vi "Linda_CORE_svi_FGV.vi"(1 "OP":T1, 5 "IN VARIANT":variant, 9 "Name in":string, 11 "error in (no error)":errorcluster, 12 "Space size":i32=1000000) -> (4 "Number of  Tuples":i32, 6 "OUT VARIANT":variant, 8 "Rd_all Array":variant[](array[variant]), 10 "Valid Op":bool, 15 "error out":errorcluster)   [LabVIEW 2015]
uses:
  LI_states.ctl
  C:/Users/Giuseppe/Downloads/LabLinda_ pakage/index_datatype.ctl
  C:/Users/Giuseppe/Downloads/LabLinda_ pakage/index_cluster.ctl
  index_datatype.ctl
  index_cluster.ctl
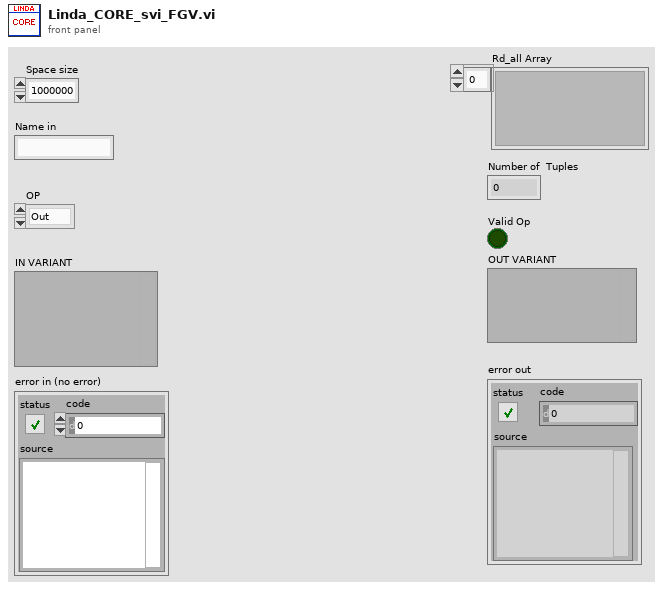
[diagram p1: front panel]
types:
  T1 = typedef "LI_states.ctl" = enum16{"Out", "In", "Rd", "Inp", "Rdp", "Init", "Cleanup", "RdAll"}
  T2 = enum16{"Init", "Read addr", "Write item", "Cleanup", "Add free", "Query Free"}
  T3 = enum32{"Invalid", "Standard", "Closed", "Hidden", "Minimized", "Maximized"}
  T4 = typedef "index_datatype.ctl" = T5[]
  T5 = typedef "index_cluster.ctl" = cluster{"Addr":i32[], "out react vi reference":refnum<vi>, "in react vi reference":refnum<vi>, "rd react vi reference":refnum<vi>, "Read_write_var":refnum<vi>}
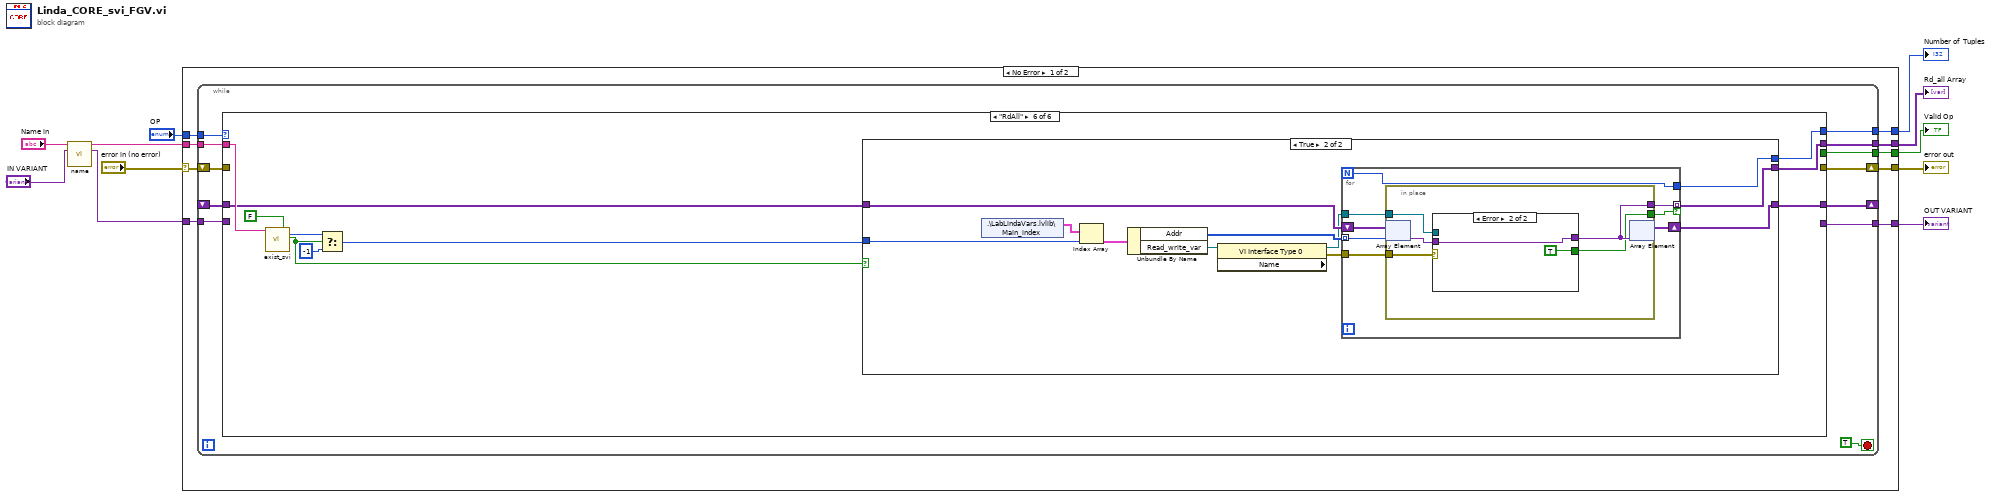
[diagram p0: block diagram]
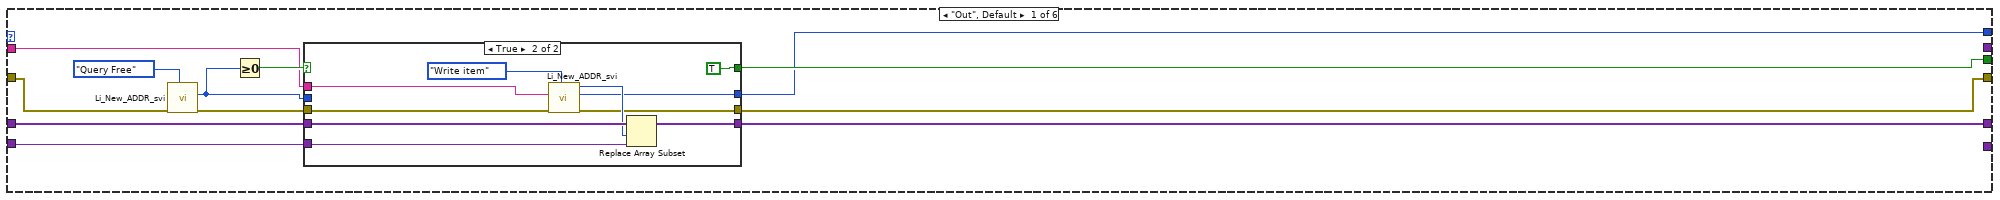
[diagram p2: hidden frame]
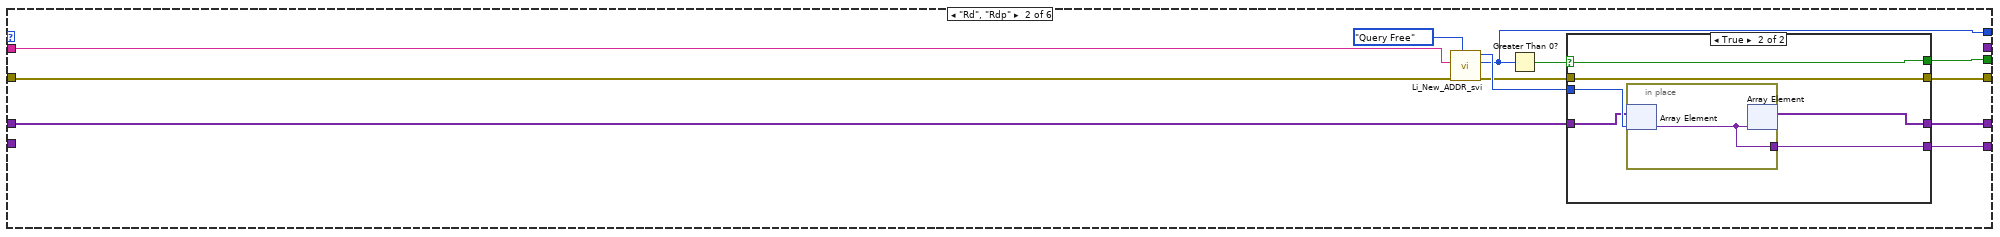
[diagram p4: hidden frame]
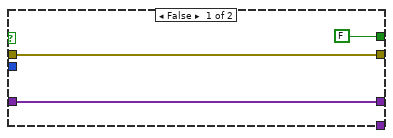
[diagram p5: hidden frame]
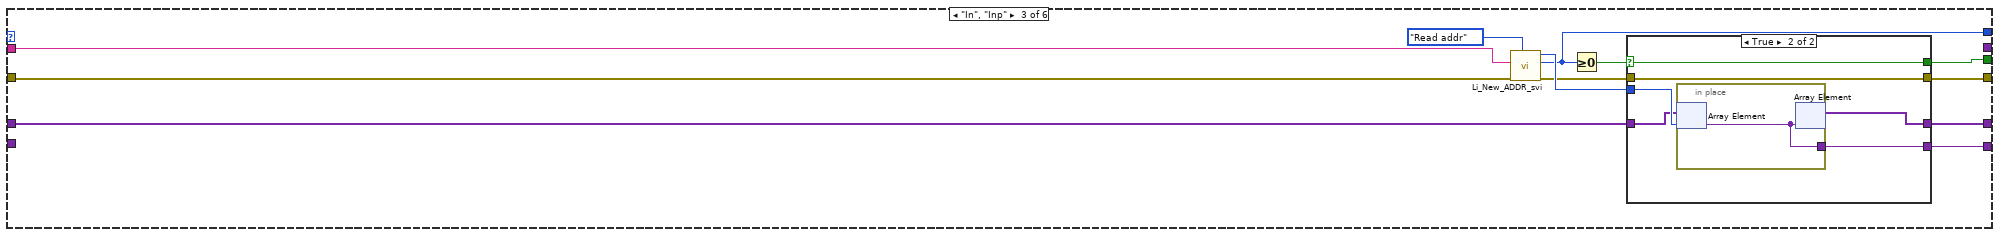
[diagram p6: hidden frame]
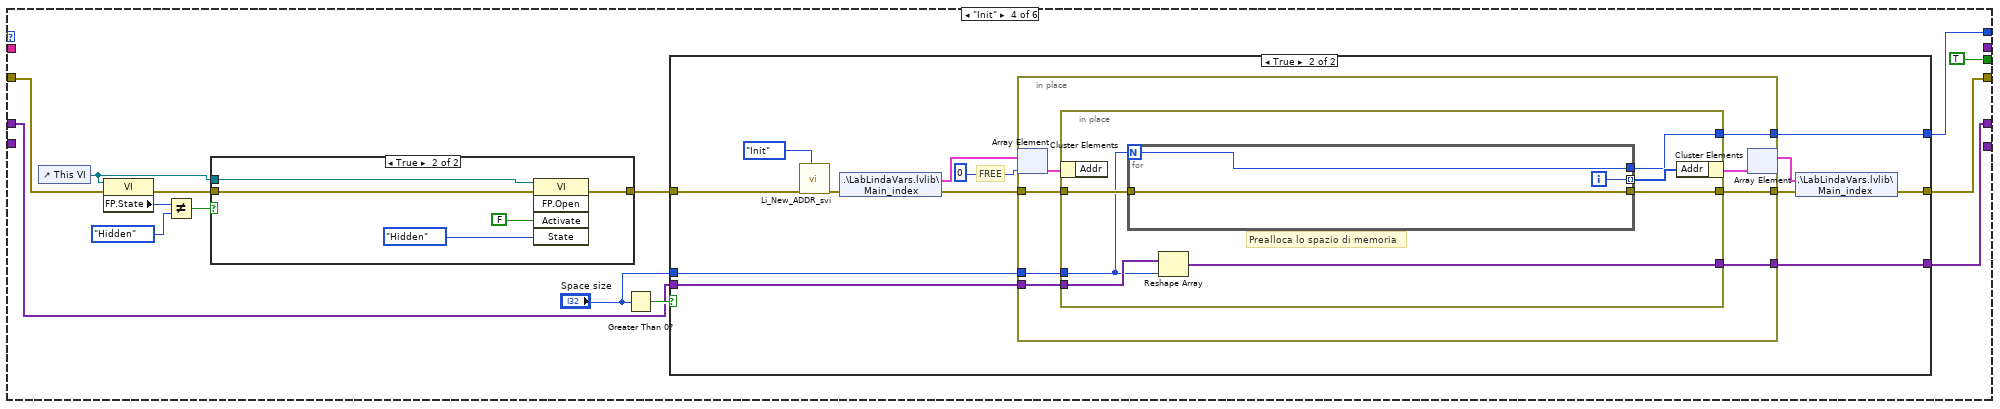
[diagram p8: hidden frame]
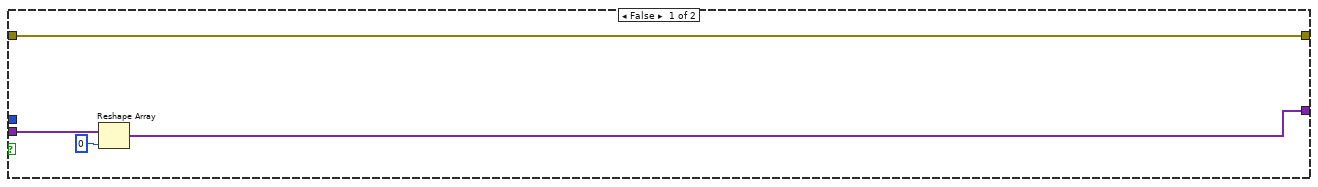
[diagram p9: hidden frame]
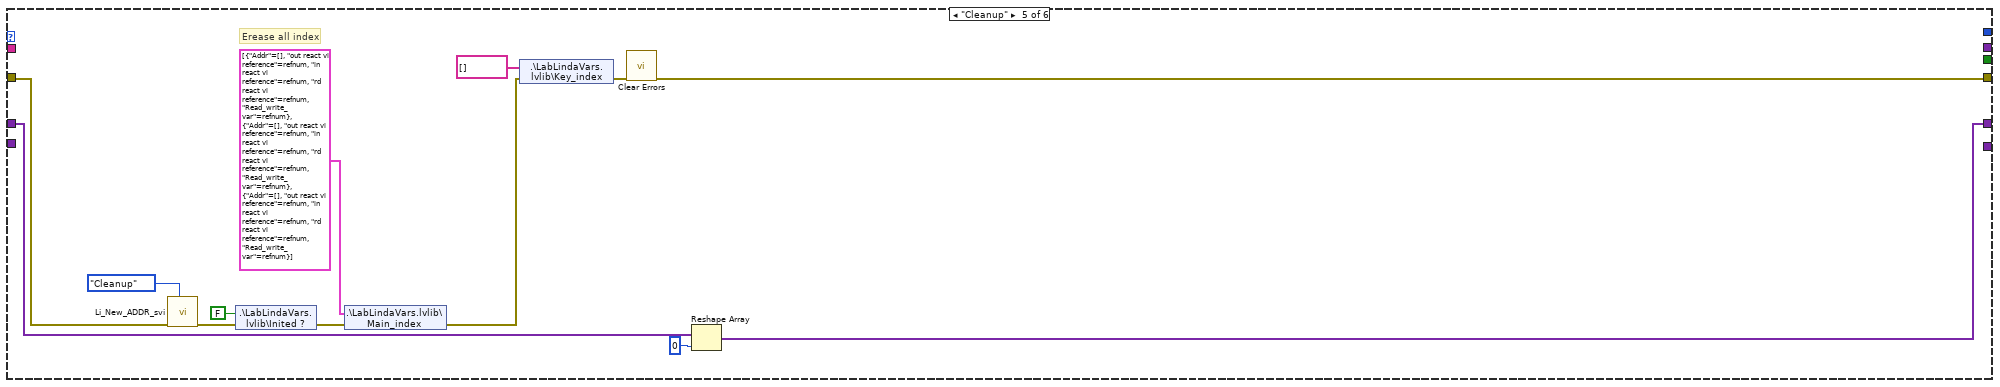
[diagram p11: hidden frame]
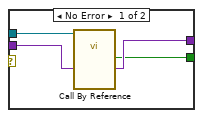
[diagram p13: hidden frame]
diagram:
  n1 = call "name.vi"("Name in"="Name in", "IN VARIANT in"="IN VARIANT") -> ("Name"=w6:string, "IN VARIANT out"=w5:variant)  [unwired: 12 in]
  n2 = case shown="No Error" "error in (no error)" {
    selector: "error in (no error)" -> [w18 w212]
    tunnel: [w20 _] -> w11
    tunnel: [w19 _] -> w10
    tunnel: [w16 w212] -> w9
    tunnel: w6 -> [w17 _]
    tunnel: "OP" -> [w15 _]
    tunnel: w5 -> [w14 _]
    tunnel: [w13 _] -> w2
    tunnel: [w12 _] -> w1
    frame No Error {
      n3 = while {
        tunnel: [w31] -> w19
        tunnel: w17 -> [w29]
        tunnel: w15 -> [w27]
        shift-right: [w28] -> w16
        shift-left: w18 -> [w30]
        tunnel: w14 -> [w26]
        tunnel: [w32] -> w20
        shift-right: [w23] -> _
        shift-left: _ -> [w25]
        tunnel: [w22] -> w13
        tunnel: [w21] -> w12
        stop <- TRUE stop-if-true
        n4 = case shown="\"RdAll\"" w27 {
          tunnel: [w38 w65 w84 w116 w159 w173] -> w23
          tunnel: w25 -> [w39 w69 w87 w103 w160 w175]
          tunnel: [w36 w66 w85 TRUE _ _] -> w31
          tunnel: [_ w67 w86 _ _ _] -> w32
          tunnel: w30 -> [w43 w70 w91 w107 w170 _]
          tunnel: w29 -> [w35 w60 w92 _ _ w177]
          tunnel: [w40 w63 w82 w115 w161 _] -> w28
          tunnel: [w34 w59 w81 w114 _ w172] -> w22
          tunnel: w26 -> [w37 _ _ _ _ _]
          tunnel: [_ _ _ _ _ w171] -> w21
          frame "Out", Default {
            n5 = call "Li_New_ADDR_svi.vi"("Op"=T2."Query Free", "error in (no error)"=w43) -> ("error out"=w41:errorcluster, "Size"=w33:i32)  [unwired: 7 in, 1 out]
            n6 = Greater Or Equal To 0?(x=w33) -> (x >= 0?=w42:bool)
            n7 = case shown="True" w42 {
              selector: w42 -> [w46 _]
              tunnel: w35 -> [_ w57]
              tunnel: w41 -> [w48 w56]
              tunnel: w39 -> [w47 w55]
              tunnel: [w47 w53] -> w38
              tunnel: [w48 w52] -> w40
              tunnel: w37 -> [_ w51]
              tunnel: [w46 TRUE] -> w36
              tunnel: [w45 w49] -> w34
              tunnel: w33 -> [w45 _]
              frame False {
              }
              frame True {
                n8 = call "Li_New_ADDR_svi.vi"("Op"=T2."Write item", "error in (no error)"=w56, "Name"=w57) -> ("error out"=w52:errorcluster, "Size"=w49:i32, "Addr"=w54:i32)  [unwired: 6 in]
                n9 = Replace Array Subset(array=w55, new element=w51, index=w54) -> (w53:variant[])
              }
            }
          }
          frame "Rd", "Rdp" {
            n10 = call "Li_New_ADDR_svi.vi"("Op"=T2."Query Free", "error in (no error)"=w70, "Name"=w60) -> ("error out"=w64:errorcluster, "Size"=w59:i32, "Addr"=w68:i32)  [unwired: 6 in]
            n11 = Greater Than 0?(x=w59) -> (x > 0?=w61:bool)
            n12 = case shown="True" w61 {
              selector: w61 -> [_ w79]
              tunnel: w69 -> [w73 w76]
              tunnel: w68 -> [_ w77]
              tunnel: [_ w74] -> w67
              tunnel: [FALSE w79] -> w66
              tunnel: [w73 w75] -> w65
              tunnel: [w72 w78] -> w63
              tunnel: w64 -> [w72 w78]
              frame False {
              }
              frame True {
                n13 = in-place {
                  in-place-border: [w80] -> w74
                  n14 = in-place-array #1(w76, w77) -> (w80:variant)
                  n15 = in-place-array #1(w80) -> (w75:variant[])  [unwired: 1 out]
                }
              }
            }
          }
          frame "In", "Inp" {
            n16 = call "Li_New_ADDR_svi.vi"("Op"=T2."Read addr", "error in (no error)"=w91, "Name"=w92) -> ("error out"=w83:errorcluster, "Size"=w81:i32, "Addr"=w88:i32)  [unwired: 6 in]
            n17 = Greater Or Equal To 0?(x=w81) -> (x >= 0?=w89:bool)
            n18 = case shown="True" w89 {
              selector: w89 -> [w94 w101]
              tunnel: w88 -> [_ w99]
              tunnel: w87 -> [w95 w98]
              tunnel: [_ w96] -> w86
              tunnel: [w94 w101] -> w85
              tunnel: [w95 w97] -> w84
              tunnel: w83 -> [w93 w100]
              tunnel: [w93 w100] -> w82
              frame False {
              }
              frame True {
                n19 = in-place {
                  in-place-border: [w102] -> w96
                  n20 = in-place-array #2(w98, w99) -> (w102:variant)
                  n21 = in-place-array #2(w102) -> (w97:variant[])  [unwired: 1 out]
                }
              }
            }
          }
          frame "Init" {
            n22 = control-ref of="This VI"() -> (w108:refnum<vi>)
            n23 = property class="VI"(reference=w108, error in=w107) -> (error out=w111:errorcluster, "FP.State"=w109:T3)  [unwired: 1 out]
            n24 = Not Equal?(x=w109, y=T3."Hidden") -> (x != y?=w112:bool)
            n25 = case shown="True" w112 {
              tunnel: [w152 w153] -> w106
              tunnel: w108 -> [_ w155]
              tunnel: w111 -> [w152 w154]
              frame False {
              }
              frame True {
                n26 = invoke class="VI" method="FP.Open"(reference=w155, error in=w154, "Activate"=FALSE ("Activate?"), "State"=T3."Hidden") -> (error out=w153:errorcluster)  [unwired: 1 in, 4 out]
              }
            }
            n27 = Greater Than 0?(x="Space size") -> (x > 0?=w104:bool)
            n28 = case shown="True" w104 {
              tunnel: [w117 w132] -> w116
              tunnel: [w120 w126] -> w115
              tunnel: [_ w125] -> w114
              tunnel: w106 -> [w120 w123]
              tunnel: "Space size" -> [_ w122]
              tunnel: w103 -> [w119 w121]
              frame False {
                n29 = Reshape Array(w119, 0 ("dimension size")) -> (w117:variant[])
              }
              frame True {
                # "FREE"
                n30 = call "Li_New_ADDR_svi.vi"("Op"=T2."Init", "error in (no error)"=w123) -> ("error out"=w124:errorcluster)  [unwired: 7 in, 2 out]
                n31 = shared-variable ".\\LabLindaVars.lvlib\\Main_index"(error in=w124) -> (w131:T4, error out=w128:errorcluster)
                n32 = in-place {
                  in-place-border: [w141] -> w132
                  in-place-border: w128 -> [w140]
                  in-place-border: [w139] -> w127
                  in-place-border: [w136] -> w125
                  in-place-border: w122 -> [w135]
                  in-place-border: w121 -> [w134]
                  n33 = in-place-array #3(w131, 0) -> (w138:T5)
                  n34 = in-place {
                    in-place-border: [w144] -> w141
                    in-place-border: w140 -> [w148]
                    in-place-border: [w147] -> w139
                    in-place-border: [w142] -> w136
                    in-place-border: w135 -> [w143]
                    in-place-border: w134 -> [w145]
                    # "Prealloca lo spazio di memoria"
                    n35 = in-place-cluster #4(w138) -> ()  [unwired: 1 out]
                    n36 = for {
                      N: w143 -> [w149]
                      tunnel: [w151] -> w146 mode=indexing
                      tunnel: w148 -> [w150]
                      tunnel: [w150] -> w147
                      tunnel: [w149] -> w142
                      i -> [w151]
                    }
                    n37 = Reshape Array(w145, w143) -> (w144:variant[])
                    n38 = in-place-cluster #4("Addr"=w146) -> (w137:T5)
                  }
                  n39 = in-place-array #3(w137) -> (w129:T4)  [unwired: 1 out]
                }
                n40 = shared-variable ".\\LabLindaVars.lvlib\\Main_index"(w129, error in=w127) -> (error out=w126:errorcluster)
              }
            }
          }
          frame "Cleanup" {
            # "Erease all index"
            n41 = call "Li_New_ADDR_svi.vi"("Op"=T2."Cleanup", "error in (no error)"=w170) -> ("error out"=w163:errorcluster)  [unwired: 7 in, 2 out]
            n42 = shared-variable ".\\LabLindaVars.lvlib\\Inited ?"(FALSE ("Inited ?"), error in=w163) -> (error out=w167:errorcluster)
            n43 = shared-variable ".\\LabLindaVars.lvlib\\Main_index"(T4 [{"Addr"=[], "out react vi reference"=refnum, "in react vi reference"=refnum, "rd react vi reference"=refnum, "Read_write_var"=refnum}, {"Addr"=[], "out react vi reference"=refnum, "in react vi reference"=refnum, "rd react vi reference"=refnum, "Read_write_var"=refnum}, {"Addr"=[], "out react vi reference"=refnum, "in react vi reference"=refnum, "rd react vi reference"=refnum, "Read_write_var"=refnum}] ("Main_index"), error in=w167) -> (error out=w165:errorcluster)
            n44 = shared-variable ".\\LabLindaVars.lvlib\\Key_index"(string[] [] ("Key_index"), error in=w165) -> (error out=w162:errorcluster)
            n45 = call <vilib>:"Clear Errors.vi"("error in (no error)"=w162) -> ("error out"=w161:errorcluster)  [unwired: 5 in, 1 out]
            n46 = Reshape Array(w160, 0 ("dimension size")) -> (w159:variant[])
          }
          frame "RdAll" {
            n47 = call "exist_svi.vi"("Name"=w177, "Create ?"=FALSE) -> ("index of element"=w180:i32, "Exist"=w174:bool)  [unwired: 14 in, 2 out]
            n48 = Select(t=w180, s=w174, f=-1) -> (s? t:f=w176:i32)
            n49 = case shown="True" w174 {
              tunnel: w176 -> [_ w191]
              tunnel: w175 -> [w181 w188]
              tunnel: [w181 w187] -> w173
              tunnel: [_ w186] -> w172
              tunnel: [_ w185] -> w171
              frame False {
              }
              frame True {
                n50 = shared-variable ".\\LabLindaVars.lvlib\\Main_index"() -> (w192:T4)  [unwired: 1 in, 1 out]
                n51 = Index Array(array=w192, index=w191) -> (element=w190:T5)
                n52 = Unbundle By Name(w190) -> ("Addr"=w189:i32[], "Read_write_var"=w183:refnum<vi>)
                n53 = property class="VI Interface Type 0" props=["Name"](reference=w183) -> (reference out=w182:refnum<vi>, error out=w184:errorcluster)  [unwired: 1 in, 1 out]
                n54 = for {
                  N -> [w197]
                  tunnel: w189 -> [w199] mode=indexing
                  tunnel: [w197] -> w186
                  tunnel: w182 -> [w196]
                  tunnel: [w195] -> w185 mode=indexing if=w193
                  tunnel: w184 -> [w194]
                  shift-right: [w198] -> w187
                  shift-left: w188 -> [w200]
                  n55 = in-place {
                    in-place-border: w196 -> [w205]
                    in-place-border: [w203] -> w195
                    in-place-border: w194 -> [w202]
                    in-place-border: [w201] -> w193
                    n56 = in-place-array #5(w200, w199) -> (w204:variant)
                    n57 = case shown="Error" w202 {
                      tunnel: w205 -> [w209 _]
                      tunnel: w204 -> [w208 w211]
                      tunnel: [w207 w211] -> w203
                      tunnel: [w206 TRUE ("Select ?")] -> w201
                      frame No Error {
                        n58 = call-by-ref "?"(reference=w209, "Vriant IN"=w208) -> ("Variant out"=w207:variant, "Select ?"=w206:bool)  [unwired: 4 in, 2 out]
                      }
                      frame Error {
                      }
                    }
                    n59 = in-place-array #5(w203) -> (w198:variant[])  [unwired: 1 out]
                  }
                }
              }
            }
          }
        }
      }
    }
    frame Error {
    }
  }
  "error out" <- w9
  "OUT VARIANT" <- w11
  "Number of  Tuples" <- w2
  "Valid Op" <- w10
  "Rd_all Array" <- w1
